vi "Re_sampling_Half_second.vi"(11 "Waveform_main":waveform(sgl)) -> (3 "Waveform":waveform(dbl))   [LabVIEW 2017]
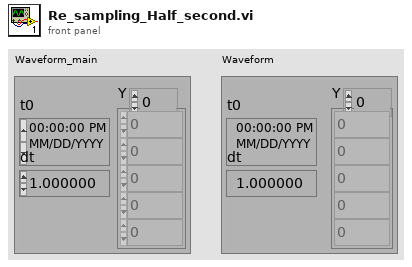
[diagram p1: front panel]
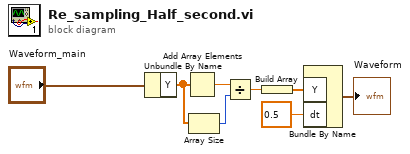
[diagram p0: block diagram]
diagram:
  n1 = Unbundle By Name("Waveform_main") -> ("Y"=w5:sgl[])
  n2 = Add Array Elements(numeric array=w5) -> (sum=w4:sgl)
  n3 = Array Size(array=w5) -> (size(s)=w3:i32)
  n4 = Divide(x=w4, y=w3) -> (x/y=w2:sgl)
  n5 = Build Array(w2) -> (w1:sgl[])
  n6 = Bundle By Name("Y"=w1, "dt"=0.5) -> (→"Waveform":waveform(sgl))  [unwired: 1 in]
